vi "Update_data_base.vi"(8 "error in (no error)":errorcluster, 9 "User id":i32, 10 "Cach":dbl, 11 "Data base":string[][](array[string])=[["Ahmed", "Hassan", "2989", "180000"], ["Ali", "Hassan", "2756", "200000"], ["Youssef", "Fady", "2020", "10"], ["Fatma", "Ali", "2003", "0"]]) -> (0 "error out":errorcluster, 3 "New Data Base":string[][](array[string]))   [LabVIEW 2025]
uses:
  <vilib>/Utility/file.llb/Write Delimited Spreadsheet (string).vi
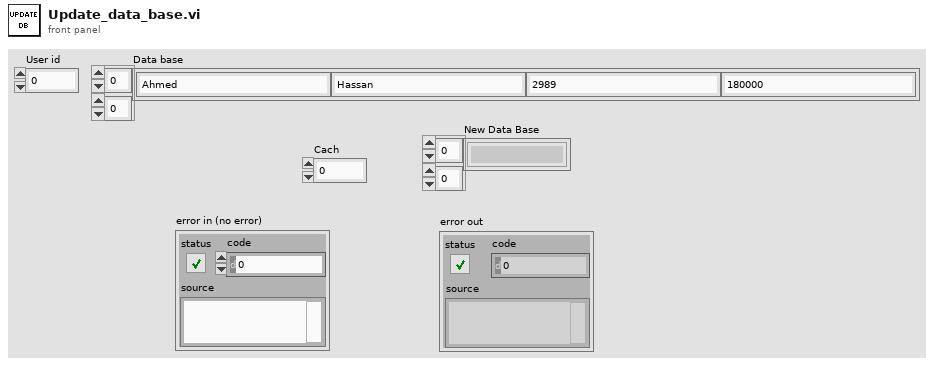
[diagram p1: front panel]
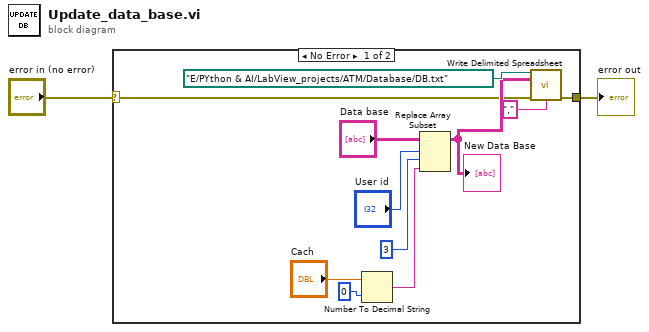
[diagram p0: block diagram]
diagram:
  n1 = case shown="No Error" "error in (no error)" {
    selector: "error in (no error)" -> [w4 w14]
    tunnel: [w3 w14] -> w1
    frame No Error {
      n2 = Number To Decimal String(number="Cach", width (-)=i16 0) -> (decimal integer string=w9:string)
      n3 = Replace Array Subset(array="Data base", new element=w9, index (row)="User id", index (col)=3) -> (w6:string[][])
      "New Data Base" <- w6
      n4 = call-poly <vilib>:"Write Delimited Spreadsheet.vi"("file path (dialog if empty)"=path "E:/PYthon & AI/LabView_projects/ATM/Database/DB.txt", "2D data"=w6, "error in (no error)"=w4, "delimiter (\\t)"="," ("delimiter (\\t)")) -> ("error out"=w3:errorcluster)  [unwired: 10 in, 1 out]
    }
    frame Error {
    }
  }
  "error out" <- w1
